vi "comms_Serial_Send_Com.vi"(8 "error in":errorcluster, 9 "Buffer Clear?":bool, 10 "Command":string, 11 "VISA resource in":refnum<visa-resource-name>) -> (0 "error out":errorcluster, 2 "Response":string, 3 "VISA resource Out":refnum<visa-resource-name>)   [LabVIEW 2018]
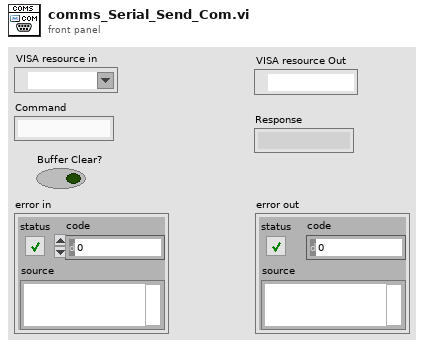
[diagram p1: front panel]
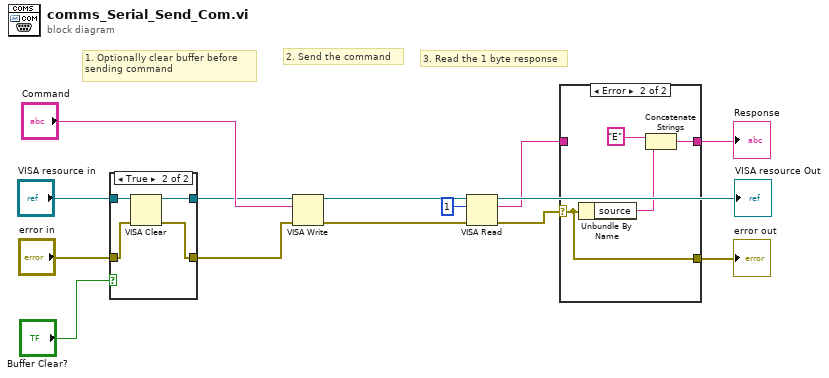
[diagram p0: block diagram]
diagram:
  # "3. Read the 1 byte response"
  # "2. Send the command"
  # "1. Optionally clear buffer before \nsending command"
  n1 = case shown="True" "Buffer Clear?" {
    tunnel: "VISA resource in" -> [w16 w20]
    tunnel: [w16 w19] -> w6
    tunnel: "error in" -> [w15 w18]
    tunnel: [w15 w17] -> w9
    frame False {
    }
    frame True {
      n2 = VISA Clear(VISA resource name=w20, error in (no error)=w18) -> (VISA resource name out=w19:refnum<visa-resource-name>, error out=w17:errorcluster)
    }
  }
  n3 = VISA Write(VISA resource name=w6, write buffer="Command", error in (no error)=w9) -> (VISA resource name out=w5:refnum<visa-resource-name>, error out=w8:errorcluster)  [unwired: 1 out]
  n4 = VISA Read(VISA resource name=w5, byte count=u32 1, error in (no error)=w8) -> (VISA resource name out=→"VISA resource Out":refnum<visa-resource-name>, read buffer=w2:string, error out=w4:errorcluster)  [unwired: 1 out]
  n5 = case shown="Error" w4 {
    selector: w4 -> [w22 w26]
    tunnel: [w22 w26] -> w3
    tunnel: w2 -> [w21 _]
    tunnel: [w21 w25] -> w1
    frame No Error {
    }
    frame Error {
      n6 = Unbundle By Name(w26) -> ("source"=w24:string)
      n7 = Concatenate Strings("E", w24) -> (w25:string)
    }
  }
  "error out" <- w3
  "Response" <- w1
